vi "All Unit Tests.vi"() -> ()   [LabVIEW 2019, in "instrument.Cryostation.lvclass"]
uses:
  instrument.Cryostation.lvclass
  <vilib>/addons/_JKI Toolkits/Caraya/classes/Assert/Assert Not Error.vi
  <vilib>/addons/_JKI Toolkits/Caraya/classes/Assert/Assert Not Equal Value_Variant.vi
  <vilib>/addons/_JKI Toolkits/Caraya/classes/Test/Test.lvclass
  <vilib>/addons/_JKI Toolkits/Caraya/classes/Assert/Assert.lvclass
panel:
  in  "address":string="130.49.180.32"
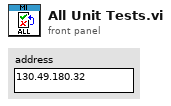
[diagram p1: front panel]
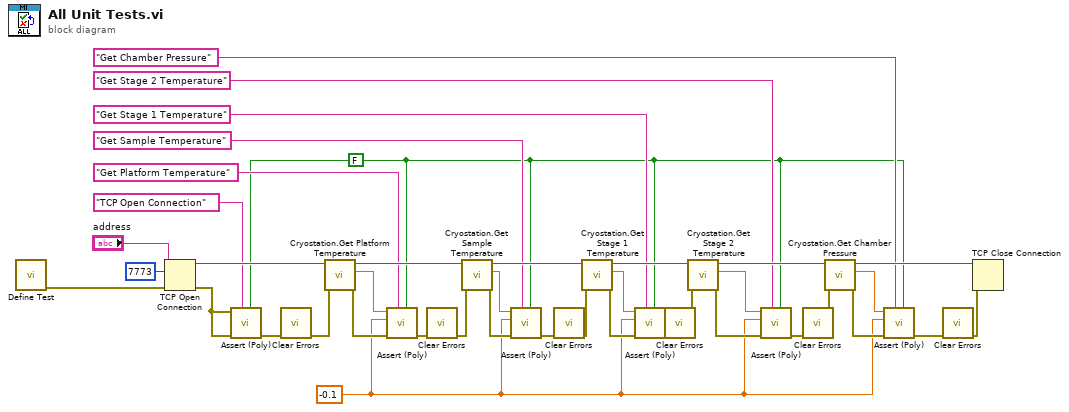
[diagram p0: block diagram]
diagram:
  w7 = FALSE ("Assert Only? (F)")
  w9 = -0.1
  n1 = call <vilib>:"Define Test.vi"() -> ("error out"=w38:errorcluster)  [unwired: 11 in]
  n2 = TCP Open Connection(address="address", remote port or service name=u16 7773, error in (no error)=w38) -> (connection ID=w36:refnum<k5>, error out=w37:errorcluster)  [unwired: 2 in]
  n3 = call-poly <vilib>:"Assert (Poly).vi"("Assert Only? (F)"=w7, "Label"="TCP Open Connection", "error in (no error)"=w37, "Not Error?"=w37) -> ("error out"=w22:errorcluster)  [unwired: 7 in]
  n4 = call <vilib>:"Clear Errors.vi"("error in (no error)"=w22) -> ("error out"=w1:errorcluster)  [unwired: 5 in, 1 out]
  n5 = call "Cryostation.Get Platform Temperature.vi"("error in (no error)"=w1, "TCP Network Connection in"=w36) -> ("error out"=w23:errorcluster, "Platform Temperature (K)"=w8:dbl, "TCP Network Connection out"=w35:refnum<k5>)  [unwired: 7 in]
  n6 = call-poly <vilib>:"Assert (Poly).vi"("Assert Only? (F)"=w7, "Label"="Get Platform Temperature", "error in (no error)"=w23, "Y"=w9, "X"=w8) -> ("error out"=w24:errorcluster)  [unwired: 6 in]
  n7 = call <vilib>:"Clear Errors.vi"("error in (no error)"=w24) -> ("error out"=w2:errorcluster)  [unwired: 5 in, 1 out]
  n8 = call "Cryostation.Get Sample Temperature.vi"("error in (no error)"=w2, "TCP Network Connection in"=w35) -> ("error out"=w11:errorcluster, "Sample Temperature (K)"=w10:dbl, "TCP Network Connection out"=w34:refnum<k5>)  [unwired: 7 in]
  n9 = call-poly <vilib>:"Assert (Poly).vi"("Assert Only? (F)"=w7, "Label"="Get Sample Temperature", "error in (no error)"=w11, "Y"=w9, "X"=w10) -> ("error out"=w25:errorcluster)  [unwired: 6 in]
  n10 = call <vilib>:"Clear Errors.vi"("error in (no error)"=w25) -> ("error out"=w6:errorcluster)  [unwired: 5 in, 1 out]
  n11 = call "Cryostation.Get Stage 1 Temperature.vi"("error in (no error)"=w6, "TCP Network Connection in"=w34) -> ("error out"=w26:errorcluster, "Stage 1 Temperature (K)"=w12:dbl, "TCP Network Connection out"=w33:refnum<k5>)  [unwired: 7 in]
  n12 = call-poly <vilib>:"Assert (Poly).vi"("Assert Only? (F)"=w7, "Label"="Get Stage 1 Temperature", "error in (no error)"=w26, "Y"=w9, "X"=w12) -> ("error out"=w27:errorcluster)  [unwired: 6 in]
  n13 = call <vilib>:"Clear Errors.vi"("error in (no error)"=w27) -> ("error out"=w5:errorcluster)  [unwired: 5 in, 1 out]
  n14 = call "Cryostation.Get Stage 2 Temperature.vi"("error in (no error)"=w5, "TCP Network Connection in"=w33) -> ("error out"=w28:errorcluster, "Stage 2 Temperature (K)"=w13:dbl, "TCP Network Connection out"=w32:refnum<k5>)  [unwired: 7 in]
  n15 = call-poly <vilib>:"Assert (Poly).vi"("Assert Only? (F)"=w7, "Label"="Get Stage 2 Temperature", "error in (no error)"=w28, "Y"=w9, "X"=w13) -> ("error out"=w14:errorcluster)  [unwired: 6 in]
  n16 = call <vilib>:"Clear Errors.vi"("error in (no error)"=w14) -> ("error out"=w4:errorcluster)  [unwired: 5 in, 1 out]
  n17 = call "Cryostation.Get Chamber Pressure.vi"("error in (no error)"=w4, "TCP Network Connection in"=w32) -> ("error out"=w29:errorcluster, "Chamber Pressure (mTorr)"=w15:dbl, "TCP Network Connection out"=w31:refnum<k5>)  [unwired: 7 in]
  n18 = call-poly <vilib>:"Assert (Poly).vi"("Assert Only? (F)"=w7, "Label"="Get Chamber Pressure", "error in (no error)"=w29, "Y"=w9, "X"=w15) -> ("error out"=w30:errorcluster)  [unwired: 6 in]
  n19 = call <vilib>:"Clear Errors.vi"("error in (no error)"=w30) -> ("error out"=w3:errorcluster)  [unwired: 5 in, 1 out]
  n20 = TCP Close Connection(connection ID=w31, error in (no error)=w3) -> ()  [unwired: 1 in, 2 out]
